vi "DI Scope Select.vi"(6 "Device Outputs in":dbl[](array[numeric]), 8 "error in":errorcluster, 9 "Device Inputs":dbl[](array[numeric]), 10 "DCM Ref":refnum<class "DCM - RT.lvclass">, 11 "DI ADC in":T1={"FIFO Indexes"={"Write"={"Capture Enable"=-1, "Capture Event"=-1, "Capture Length"=-1, "DI ADC 1 Select"=-1, "DI ADC 2 Select"=-1, "DI ADC 3 Select"=-1, "DI ADC 4 Select"=-1}, "Read"={"Capture dt [s]"=-1}}, "DI ADC Data"={"Output Array"=[], "New Data"=FALSE}, "Waveform Data"=[], "Waveform Session"=refnum}) -> (0 "error out":errorcluster, 3 "DI ADC out":T1={"FIFO Indexes"={"Write"={"Capture Enable"=-1, "Capture Event"=-1, "Capture Length"=-1, "DI ADC 1 Select"=0, "DI ADC 2 Select"=0, "DI ADC 3 Select"=-1, "DI ADC 4 Select"=-1}, "Read"={"Capture dt [s]"=-1}}, "DI ADC Data"={"Output Array"=[], "New Data"=FALSE}, "Waveform Data"=[], "Waveform Session"=refnum}, 4 "Device Outputs out":dbl[](array[numeric]))   [LabVIEW 2016, in "DCM Engine.lvlib"]
uses:
  DCM Engine.lvlib
  Shared/Types/DI Scope.ctl
  <vilib>/NI Veristand/Custom Device Waveform API/Multiple Waveforms Write (DBL)/Multiple Waveforms Write (DBL).lvclass
  <vilib>/NI Veristand/Custom Device API/Waveform Data Reference.ctl
  Built/DCM Classes Packed/Pharlap/C/DCM-Classes.lvlibp/DCM/Rev0/RT/DCM - RT.lvclass
  Built/DCM Classes Packed/Pharlap/C/DCM-Classes.lvlibp/DCM/Rev0/RT/DI - ADC Select.ctl
  Built/DCM Classes Packed/Pharlap/C/DCM-Classes.lvlibp/1abvi3w/vi.lib/Powertrain Controls/Device Drivers/DCM/Rev0/FPGA/DI - ADC Signals.ctl
  <vilib>/NI Veristand/Custom Device Waveform API/Multiple Waveforms Write (DBL)/NI VeriStand - Close Multiple Waveforms Write Session (DBL).vi
  <vilib>/NI Veristand/Custom Device Waveform API/Multiple Waveforms Write (DBL)/NI VeriStand - Open Multiple Waveforms Write Session (DBL).vi
  Built/DCM Classes Packed/Pharlap/C/DCM-Classes.lvlibp/DCM/DI/RT/DCM - RT - DI.lvlib
  Built/DCM Classes Packed/Pharlap/C/DCM-Classes.lvlibp/1abvi3w/vi.lib/Powertrain Controls/Device Drivers/DCM/Rev0/FPGA/DCM - FPGA.lvlib
  <vilib>/NI Veristand/Custom Device Waveform API/NI_VS Custom Device Waveform API.lvlib
  DCM Shared.lvlib
  <vilib>/NI VeriStand/Custom Device API/Custom Device API.lvlib
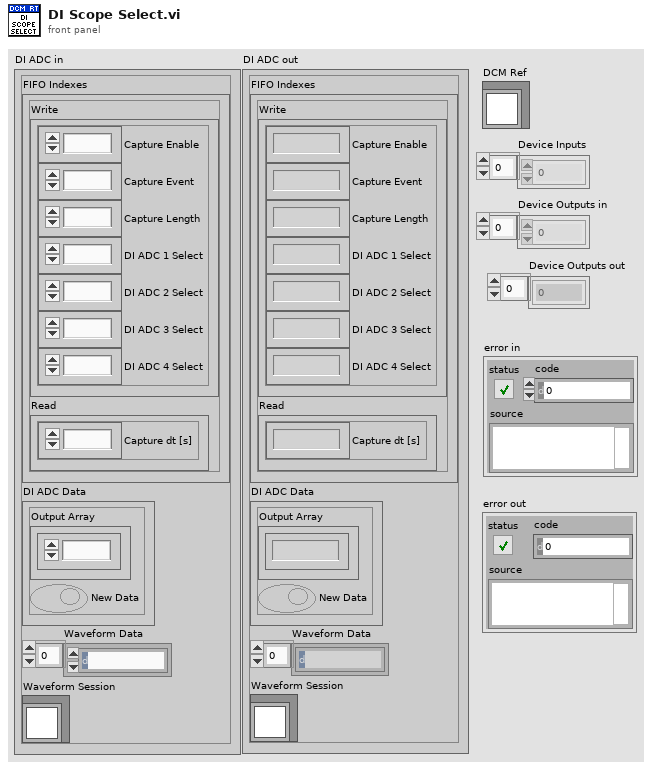
[diagram p1: front panel]
types:
  T1 = typedef "DCM Shared.lvlib/DI Scope.ctl" = cluster{"FIFO Indexes":cluster{"Write":cluster{"Capture Enable":i32, "Capture Event":i32, "Capture Length":i32, "DI ADC 1 Select":i32, "DI ADC 2 Select":i32, "DI ADC 3 Select":i32, "DI ADC 4 Select":i32}, "Read":cluster{"Capture dt [s]":i32}}, "DI ADC Data":cluster{"Output Array":sgl[][], "New Data":bool}, "Waveform Data":T2[], "Waveform Session":refnum<class "Multiple Waveforms Write (DBL).lvclass">}
  T2 = typedef "Custom Device API.lvlib/Waveform Data Reference.ctl" = i32
  T3 = typedef "DCM-Classes.lvlibp/DCM - RT.lvclass/DI - ADC Select.ctl" = cluster{"DI ADC 1":T4, "DI ADC 2":T4, "DI ADC 3":T4, "DI ADC 4":T4}
  T4 = typedef "DCM-Classes.lvlibp/DCM - FPGA.lvlib/DI - ADC Signals.ctl" = enum8{"I LS A1/A5", "I LS A2/A6", "I LS A3/A7", "I LS A4", "I LS A8/PumpA", "V PZ A1", "V PZ A2", "V PZ A3", "V PZ A4", "V S A1", "V S A2", "V S A3", "V S A4", "V S A5", "V S A6", "V S A7", "V S A8", "V Pump A", "V Secondary A1A2", "V Secondary A3A4", "V Ext HV A", "------------------------ ", "I LS B1/B5", "I LS B2/B6", "I LS B3/B7", "I LS B4", "I LS B8/PumpB", "V PZ B1", "V PZ B2", "V PZ B3", "V PZ B4", "V S B1", "V S B2", "V S B3", "V S B4", "V S B5", "V S B6", "V S B7", "V S B8", "V Pump B", "V Secondary B1B2", "V Secondary B3B4", "V Ext HV B", "-------------------------  ", "AI 1", "AI 2", "AI 3", "AI 4", "AI 5", "AI 6", "AI 7", "AI 8", "AI 9", "AI 10", "AI 11", "AI 12", "-------------------------   ", "V DRVP"}
  T5 = cluster{"Capture Enable":i32, "Capture Event":i32, "Capture Length":i32, "DI ADC 1 Select":i32, "DI ADC 2 Select":i32, "DI ADC 3 Select":i32, "DI ADC 4 Select":i32}
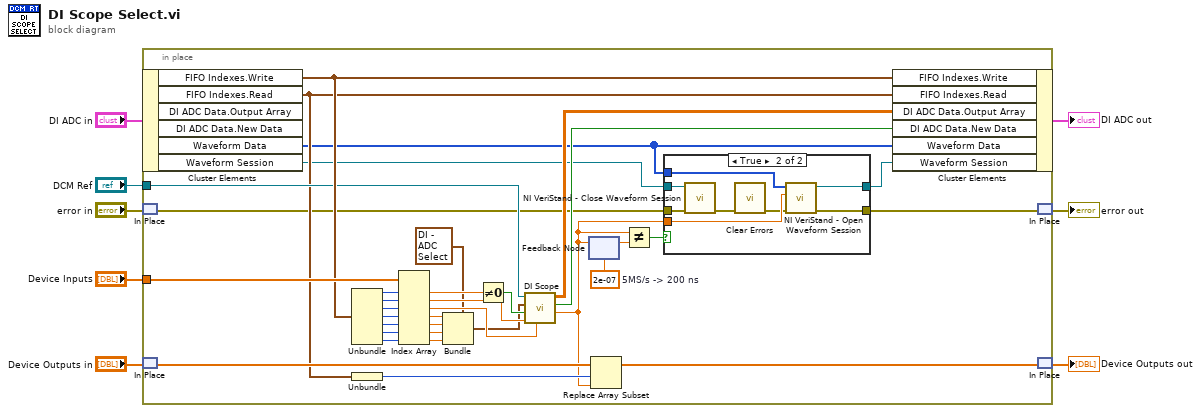
[diagram p0: block diagram]
diagram:
  n1 = in-place {
    in-place-border: "Device Inputs" -> [w43]
    in-place-border: "DCM Ref" -> [w34]
    w10 = 2e-07  # 5MS/s -> 200 ns
    n2 = in-place-cluster #1("DI ADC in") -> ("FIFO Indexes.Write"=w40:T5, "FIFO Indexes.Read"=w20:cluster{"Capture dt [s]":i32}, "Waveform Data"=w11:T2[], "Waveform Session"=w13:refnum<class "Multiple Waveforms Write (DBL).lvclass">)  [unwired: 2 out]
    n3 = in-place-match #2("error in") -> (w16:errorcluster)
    n4 = in-place-match #3("Device Outputs in") -> (w23:dbl[])
    n5 = Unbundle(w40) -> ("Capture Enable"=w42:i32, "Capture Event"=w41:i32, "Capture Length"=w29:i32, "DI ADC 1 Select"=w30:i32, "DI ADC 2 Select"=w31:i32, "DI ADC 3 Select"=w32:i32, "DI ADC 4 Select"=w33:i32)
    n6 = Unbundle(w20) -> ("Capture dt [s]"=w21:i32)
    n7 = Index Array(array=w43, index #1=w42, index #2=w41, index #3=w29, index #4=w30, index #5=w31, index #6=w32, index #7=w33) -> (element #1=w37:dbl, element #2=w35:dbl, element #3=w24:dbl, element #4=w28:dbl, element #5=w27:dbl, element #6=w26:dbl, element #7=w25:dbl)
    n8 = Bundle(cluster=T3 {"DI ADC 1"=enum."I LS A1/A5", "DI ADC 2"=enum."I LS A1/A5", "DI ADC 3"=enum."I LS A1/A5", "DI ADC 4"=enum."I LS A1/A5"} ("Channel Select"), "DI ADC 1"=w28, "DI ADC 2"=w27, "DI ADC 3"=w26, "DI ADC 4"=w25) -> (w18:T3)
    n9 = Not Equal To 0?(x=w37) -> (x != 0?=w36:bool)
    n10 = call "DI Scope.vi"("DI Scope Length [s]"=w24, "DI Scope Event"=w35, "DI Scope Capture"=w36, "Channel Select"=w18, "DCM Reference"=w34) -> ("dT [s]"=w14:sgl, "New Data"=w38:bool, "Data"=w39:sgl[][])  [unwired: 3 in, 1 out]
    n11 = feedback #4(w10) -> (w17:dbl)
    n12 = feedback-in #4(w14) -> ()
    n13 = Replace Array Subset(array=w23, new element=w14, index=w21) -> (w22:dbl[])
    n14 = Not Equal?(x=w14, y=w17) -> (x != y?=w9:bool)
    n15 = case shown="True" w9 {
      tunnel: w13 -> [w44 w53]
      tunnel: w16 -> [w45 w52]
      tunnel: [w45 w50] -> w15
      tunnel: [w44 w49] -> w12
      tunnel: w14 -> [_ w48]
      tunnel: w11 -> [_ w47]
      frame False {
      }
      frame True {
        n16 = call-poly <vilib>:"NI VeriStand - Close Waveform Session.vi"("error in (no error)"=w52, "Multiple Waveforms Write Session (DBL)"=w53) -> ("error out"=w51:errorcluster)  [unwired: 9 in]
        n17 = call <vilib>:"Clear Errors.vi"("error in (no error)"=w51) -> ("error out"=w46:errorcluster)  [unwired: 5 in, 1 out]
        n18 = call-poly <vilib>:"NI VeriStand - Open Waveform Session.vi"("error in (no error)"=w46, "dt"=w48, "DBL Waveform Data References"=w47) -> ("error out"=w50:errorcluster, "Multiple Waveforms Write Session (DBL)"=w49:refnum<class "Multiple Waveforms Write (DBL).lvclass">)  [unwired: 7 in]
      }
    }
    n19 = in-place-cluster #1("FIFO Indexes.Write"=w40, "FIFO Indexes.Read"=w20, "DI ADC Data.Output Array"=w39, "DI ADC Data.New Data"=w38, "Waveform Data"=w11, "Waveform Session"=w12) -> (→"DI ADC out":T1)
    n20 = in-place-match #2(w15) -> (→"error out":errorcluster)
    n21 = in-place-match #3(w22) -> (→"Device Outputs out":dbl[])
  }
